vi "CheckIfGObjectMatches.vi"(8 "error in (no error)":errorcluster, 10 "GObj Refnum":refnum<vi>, 11 "Control Layout in":refnum<class "Tree Control Layout.lvclass">) -> (0 "error out":errorcluster, 2 "compatible?":bool)   [LabVIEW 2010, in "NI_SE_Front Panel Layout.lvlib" / "Tree Control Layout.lvclass"]
uses:
  Tree Control Layout.lvclass
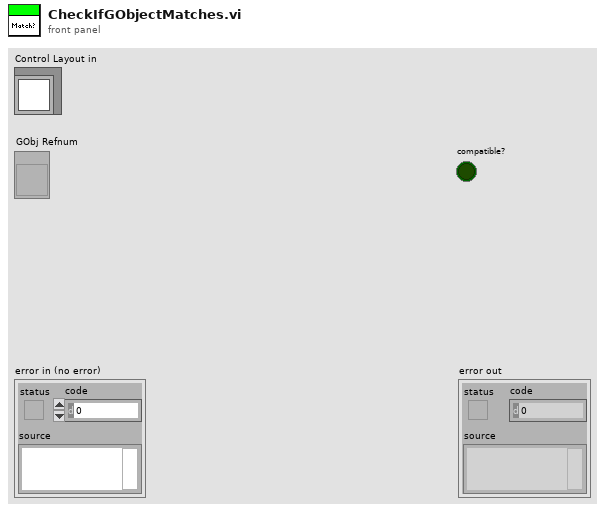
[diagram p1: front panel]
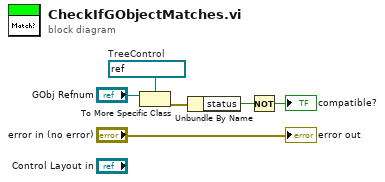
[diagram p0: block diagram]
diagram:
  w4 = refnum<vi> refnum  # TreeControl
  n1 = To More Specific Class(target class=w4, reference="GObj Refnum") -> (error out=w3:errorcluster)  [unwired: 1 in, 1 out]
  n2 = Unbundle By Name(w3) -> ("status"=w1:bool)
  n3 = Not(x=w1) -> (.not. x?=→"compatible?":bool)
  "error out" <- "error in (no error)"
